vi "DetachNewPackets.vi"(6 "SampleLen":i32, 7 "SamplesInPacketNrLen":i32, 8 "ErrorIn":errorcluster, 9 "PacketsNum":u32, 10 "PacketsIn":T1[](array[typedef]) {"MeasurementConfig"."Resolution[b]" min=4 max=16 step=1; "MeasurementConfig"."Frequency" min=1 max=10000000 step=1}, 11 "FrameIn":string) -> (0 "ErrorOut":errorcluster, 2 "PacketsOut":T1[](array[typedef]) {"MeasurementConfig"."Resolution[b]" min=4 max=16 step=1; "MeasurementConfig"."Frequency" min=1 max=10000000 step=1}, 3 "FrameOut":string)   [LabVIEW 2016]
doc: "Convert and append packets into a frame (string)."
uses:
  FallSensor/Packet.ctl
  FallSensor/Sample.ctl
  FallSensor/Reading.ctl
  FallSensor/MeasurementConfig.ctl
  FallSensor/Measurement/AccelFSRange.ctl
  FallSensor/Measurement/GyroFSRange.ctl
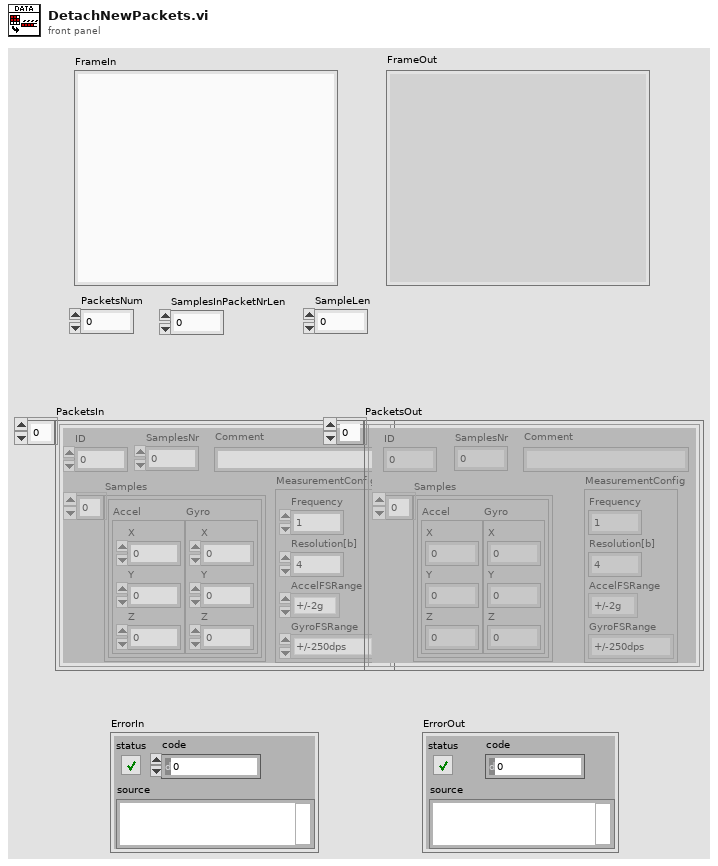
[diagram p1: front panel]
types:
  T1 = typedef "Packet.ctl" = cluster{"ID":u32, "SamplesNr":u32, "Samples":T2[], "MeasurementConfig":T4, "Comment":string}
  T2 = typedef "Sample.ctl" = cluster{"Accel":T3, "Gyro":T3}
  T3 = typedef "Reading.ctl" = cluster{"X":i16, "Y":i16, "Z":i16}
  T4 = typedef "MeasurementConfig.ctl" = cluster{"Frequency":u32, "Resolution[b]":u32, "AccelFSRange":T5, "GyroFSRange":T6}
  T5 = typedef "AccelFSRange.ctl" = enum16{"+/-2g", "+/-4g", "+/-8g", "+/-16g"}
  T6 = typedef "GyroFSRange.ctl" = enum16{"+/-250dps", "+/-500dps", "+/-1000dps", "+/-2000dps"}
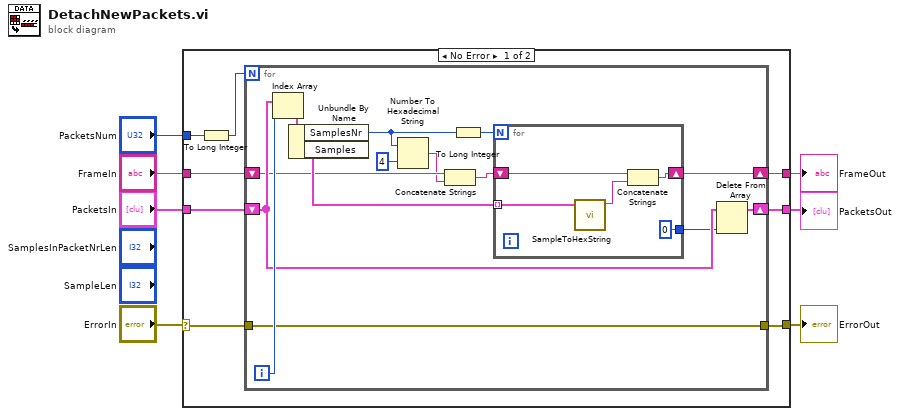
[diagram p0: block diagram]
diagram:
  n1 = case shown="No Error" "ErrorIn" {
    selector: "ErrorIn" -> [w9 w37]
    tunnel: [w8 w37] -> w6
    tunnel: "PacketsNum" -> [w15 _]
    tunnel: "FrameIn" -> [w13 w36]
    tunnel: "PacketsIn" -> [w12 w35]
    tunnel: [w11 w36] -> w2
    tunnel: [w10 w35] -> w1
    frame No Error {
      n2 = To Long Integer(number=w15) -> (32bit integer=w14:i32)
      n3 = for {
        N: w14 -> [_]
        shift-right: [w28] -> w11
        shift-left: w13 -> [w19]
        shift-right: [w22] -> w10
        shift-left: w12 -> [w24]
        tunnel: w9 -> [w21]
        tunnel: [w21] -> w8
        i -> [w26]
        n4 = Index Array(array=w24, index=w26) -> (element=w27:T1)
        n5 = Unbundle By Name(w27) -> ("SamplesNr"=w17:u32, "Samples"=w25:T2[])
        n6 = Number To Hexadecimal String(1:i16 4 ("width (-)"), 2:w17) -> (0:w18:string)
        n7 = Concatenate Strings(w19, w18) -> (w20:string)
        n8 = To Long Integer(number=w17) -> (32bit integer=w29:i32)
        n9 = for {
          N: w29 -> [_]
          shift-right: [w31] -> w28
          shift-left: w20 -> [w33]
          tunnel: w25 -> [w34] mode=indexing
          tunnel: [0 ("index")] -> w23
          n10 = call "SampleToHexString.vi"("Sample"=w34) -> ("StringOut"=w32:string)  [unwired: 10 in]
          n11 = Concatenate Strings(w33, w32) -> (w31:string)
        }
        n12 = Delete From Array(array=w24, index=w23) -> (array with subset deleted=w22:T1[])  [unwired: 1 in, 1 out]
      }
    }
    frame Error {
    }
  }
  "PacketsOut" <- w1
  "FrameOut" <- w2
  "ErrorOut" <- w6
